vi "Create.vi"(7 "Max Errors (200)":i32=200) -> (2 "MultiErrors out":refnum<class "MultiErrors.lvclass">)   [LabVIEW 2020, in "VolatusErrorUtilities.lvlib" / "MultiErrors.lvclass"]
uses:
  MultiErrors.lvclass
  MultiError.ctl
  MultiErrors.lvclass/MultiErrors.ctl
  VolatusErrorUtilities.lvlib
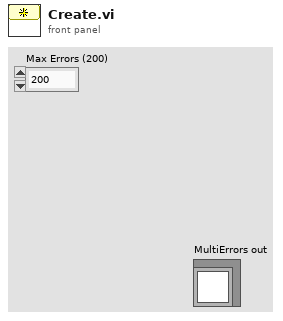
[diagram p1: front panel]
types:
  T1 = typedef "VolatusErrorUtilities.lvlib/MultiError.ctl" = cluster{"Context":string[], "Message":string, "Code":i32, "Call Chain":string[]}
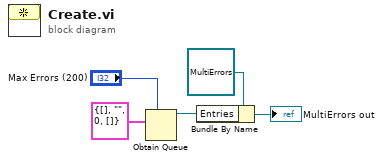
[diagram p0: block diagram]
diagram:
  n1 = Obtain Queue(max queue size (-1, unlimited)="Max Errors (200)", element data type=T1 {"Context"=[], "Message"="", "Code"=0, "Call Chain"=[]} ("MultiError Entry")) -> (queue out=w1:refnum<queue>)  [unwired: 3 in, 2 out]
  n2 = Bundle By Name(cluster=refnum<class "MultiErrors.lvclass"> refnum ("MultiErrors in"), "Entries"=w1) -> (→"MultiErrors out":refnum<class "MultiErrors.lvclass">)
